vi "Replase ALR_ON_OFF.vi"(6 "Message":string, 8 "error in":errorcluster, 9 "Action":string, 10 "ALR_Names":string[](array[string]), 11 "Alarms_in":T1) -> (0 "error out":errorcluster, 3 "ALR_ON_OFF out":T1)   [LabVIEW 2019, in "Alarms.lvlib"]
uses:
  Alarms.lvlib
  Ctl/Alarms.ctl
  Ctl/ALR_defs.ctl
  Ctl/ALRs_State.ctl
  Ctl/ALR_ON_OFF.ctl
  Ctl/ALR_Parameters.ctl
  Ctl/ALR code.ctl
  Ctl/ALR type.ctl
  <vilib>/JDP Science/JSONtext/Find Multiple Items.vi
  <vilib>/JDP Science/JSONtext/String Subset.vi
  <vilib>/JDP Science/JSONtext/support/Strip Quotes and Unescape.vi
  <vilib>/JDP Science/JSONtext/Parsing/Parse Full Path or Item Name.vi
  <vilib>/JDP Science/JSONtext/Offset/Find Item Locations by Path.vi
  <vilib>/JDP Science/JSONtext/support/Unescape JSON string.vi
  <vilib>/JDP Science/JSONtext/Get Array Elements.vi
  Userlib.lvlib
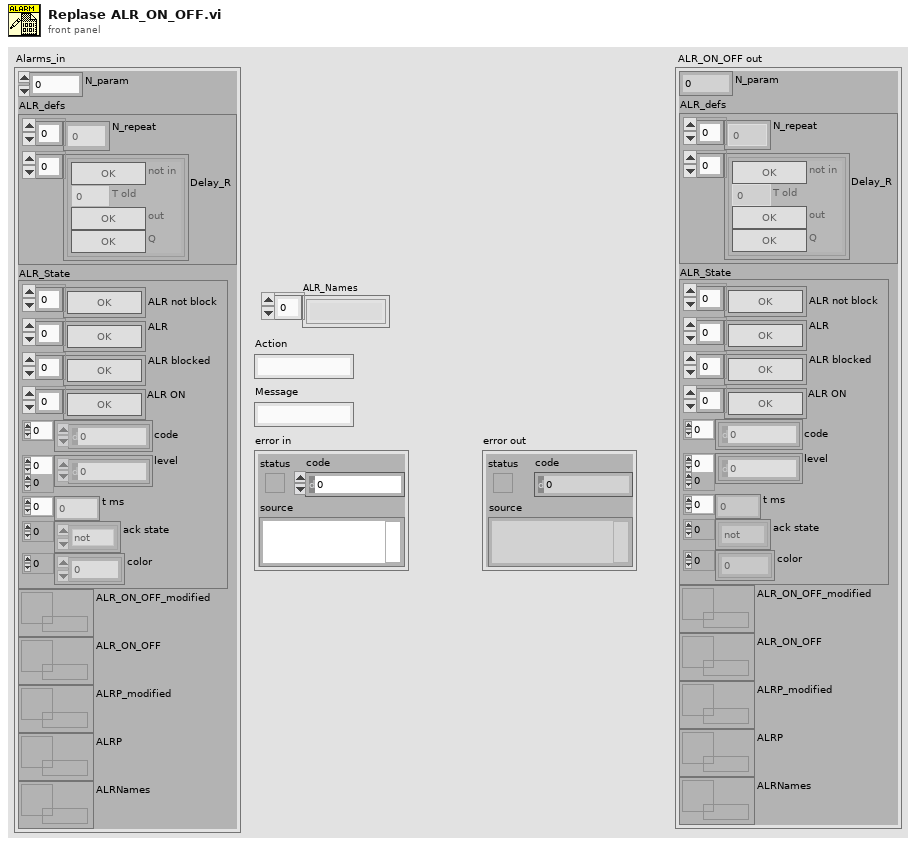
[diagram p1: front panel]
types:
  T1 = typedef "Alarms.lvlib/Alarms.ctl" = cluster{"N_param":i32, "ALR_defs":T2, "ALR_State":T3, "ALR_ON_OFF_modified":refnum<data-value>, "ALR_ON_OFF":refnum<data-value>, "ALRP_modified":refnum<data-value>, "ALRP":refnum<data-value>, "ALRNames":refnum<data-value>}
  T2 = typedef "Alarms.lvlib/ALR_defs.ctl" = cluster{"N_repeat":u32[], "Delay_R":cluster{"not in":bool, "T old":u32, "out":bool, "Q":bool}[]}
  T3 = typedef "Alarms.lvlib/ALRs_State.ctl" = cluster{"ALR not block":bool[], "ALR":bool[], "ALR blocked":bool[], "ALR ON":bool[], "code":i32[], "level":i32[][], "t ms":u32[], "ack state":enum32{"not", "tripped", "reset", "ack"}[], "color":u32[]}
  T4 = typedef "Alarms.lvlib/ALR_ON_OFF.ctl" = cluster{"ALR_ON":bool[], "ALR_OFF":bool[], "ALR_reset":bool[], "ALR_check":bool[], "ALR_block":bool[], "ALR_Ack":bool[]}
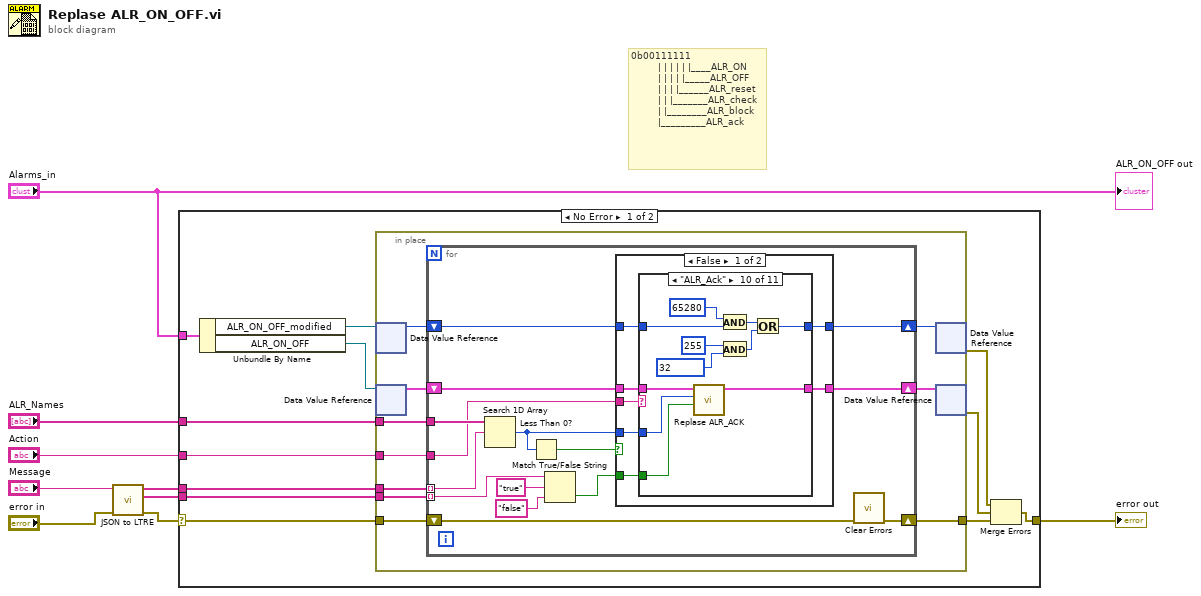
[diagram p0: block diagram]
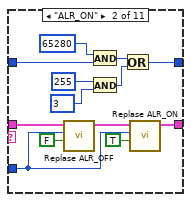
[diagram p3: hidden frame]
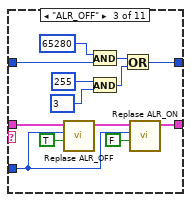
[diagram p4: hidden frame]
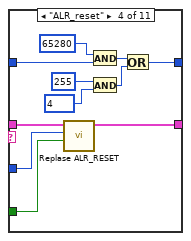
[diagram p5: hidden frame]
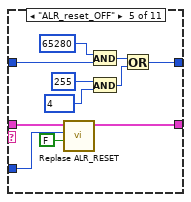
[diagram p6: hidden frame]
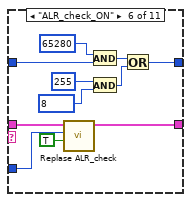
[diagram p7: hidden frame]
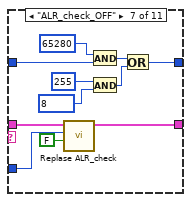
[diagram p8: hidden frame]
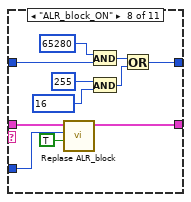
[diagram p9: hidden frame]
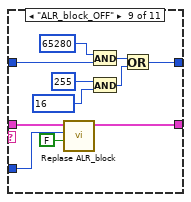
[diagram p10: hidden frame]
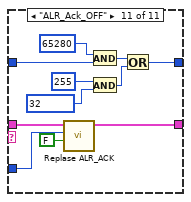
[diagram p11: hidden frame]
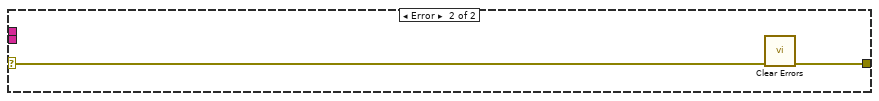
[diagram p13: hidden frame]
diagram:
  # "0b00111111\n         | | | | | |____ALR_ON\n         | | | | |_____ALR_OFF\n         | | | |______ALR_reset\n         | | |_______ALR_check\n         | |________ALR_block\n         |_________ALR_ack"
  n1 = call "JSON to LTRE.vi"("error in (no error)"="error in", "JSON Data In"="Message") -> ("error out"=w5:errorcluster, "values"=w4:string[], "names"=w3:string[])  [unwired: 7 in]
  n2 = case shown="No Error" w5 {
    selector: w5 -> [w21 w173]
    tunnel: w4 -> [w16 _]
    tunnel: [w18 w172] -> w9
    tunnel: w3 -> [w17 _]
    tunnel: "Action" -> [w15 _]
    tunnel: "Alarms_in" -> [w14 _]
    tunnel: "ALR_Names" -> [w11 _]
    frame No Error {
      n3 = Unbundle By Name(w14) -> ("ALR_ON_OFF_modified"=w13:refnum<data-value>, "ALR_ON_OFF"=w12:refnum<data-value>)
      n4 = in-place {
        in-place-border: w21 -> [w29]
        in-place-border: [w28] -> w19
        in-place-border: w17 -> [w27]
        in-place-border: w16 -> [w26]
        in-place-border: w15 -> [w25]
        in-place-border: w11 -> [w22]
        n5 = in-place-dvr #1(w13) -> (w24:u16)  [unwired: 1 out]
        n6 = in-place-dvr #2(w12) -> (w31:T4)  [unwired: 1 out]
        n7 = for {
          shift-right: [w45] -> w30
          shift-left: w31 -> [w46]
          tunnel: w27 -> [w44] mode=indexing
          tunnel: w22 -> [w43]
          tunnel: w26 -> [w34] mode=indexing
          shift-right: [w41] -> w28
          shift-left: w29 -> [w33]
          tunnel: w25 -> [w40]
          shift-right: [w38] -> w23
          shift-left: w24 -> [w39]
          n8 = Search 1D Array(1D array=w43, element=w44) -> (index of element=w42:i32)  [unwired: 1 in]
          n9 = Less Than 0?(x=w42) -> (x < 0?=w32:bool)
          n10 = Match True/False String(2:"false" ("false string"), 3:"true" ("true string"), 4:w34) -> (0:w35:bool)  [unwired: 1 out]
          n11 = case shown="False" w32 {
            tunnel: w46 -> [w53 w171]
            tunnel: [w52 w171] -> w45
            tunnel: w42 -> [w51 _]
            tunnel: w35 -> [w49 _]
            tunnel: w40 -> [w50 _]
            tunnel: w39 -> [w48 w170]
            tunnel: [w47 w170] -> w38
            frame False {
              n12 = case shown="\"ALR_Ack\"" w50 {
                tunnel: w53 -> [w55 w65 w79 w92 w103 w114 w125 w136 w147 w158 w169]
                tunnel: [w55 w68 w76 w91 w102 w113 w124 w135 w146 w157 w168] -> w52
                tunnel: w51 -> [_ w64 w78 w90 w100 w111 w122 w133 w144 w156 w166]
                tunnel: w49 -> [_ _ _ w89 _ _ _ _ _ w155 _]
                tunnel: w48 -> [w54 w56 w69 w83 w93 w104 w115 w126 w137 w149 w159]
                tunnel: [w54 w57 w70 w84 w94 w105 w116 w127 w138 w148 w160] -> w47
                frame "UNDEFINED", Default {
                }
                frame "ALR_ON" {
                  n13 = call "Replase ALR_OFF.vi"("ALR_OFF"=FALSE ("ALR_ON"), "N"=w64, "ALR_ON_OFF in"=w65) -> ("ALR_ON_OFF out"=w63:T4)  [unwired: 8 in]
                  n14 = And(x=u16 65280, y=w56) -> (x .and. y?=w62:u16)
                  n15 = And(x=u16 255, y=u16 3 ("modified (0)")) -> (x .and. y?=w61:u16)
                  n16 = Or(x=w62, y=w61) -> (x .or. y?=w57:u16)
                  n17 = call "Replase ALR_ON.vi"("ALR_ON"=TRUE, "N"=w64, "ALR_ON_OFF in"=w63) -> ("ALR_ON_OFF out"=w68:T4)  [unwired: 8 in]
                }
                frame "ALR_OFF" {
                  n18 = call "Replase ALR_OFF.vi"("ALR_OFF"=TRUE ("ALR_ON"), "N"=w78, "ALR_ON_OFF in"=w79) -> ("ALR_ON_OFF out"=w77:T4)  [unwired: 8 in]
                  n19 = And(x=u16 65280, y=w69) -> (x .and. y?=w75:u16)
                  n20 = And(x=u16 255, y=u16 3 ("modified (0)")) -> (x .and. y?=w74:u16)
                  n21 = Or(x=w75, y=w74) -> (x .or. y?=w70:u16)
                  n22 = call "Replase ALR_ON.vi"("ALR_ON"=FALSE, "N"=w78, "ALR_ON_OFF in"=w77) -> ("ALR_ON_OFF out"=w76:T4)  [unwired: 8 in]
                }
                frame "ALR_reset" {
                  n23 = call "Replase ALR_RESET.vi"("ALR_RST"=w89, "N"=w90, "ALR_ON_OFF in"=w92) -> ("ALR_ON_OFF out"=w91:T4)  [unwired: 8 in]
                  n24 = And(x=u16 65280, y=w83) -> (x .and. y?=w88:u16)
                  n25 = And(x=u16 255, y=u16 4 ("modified (0)")) -> (x .and. y?=w87:u16)
                  n26 = Or(x=w88, y=w87) -> (x .or. y?=w84:u16)
                }
                frame "ALR_reset_OFF" {
                  n27 = call "Replase ALR_RESET.vi"("ALR_RST"=FALSE, "N"=w100, "ALR_ON_OFF in"=w103) -> ("ALR_ON_OFF out"=w102:T4)  [unwired: 8 in]
                  n28 = And(x=u16 65280, y=w93) -> (x .and. y?=w99:u16)
                  n29 = And(x=u16 255, y=u16 4 ("modified (0)")) -> (x .and. y?=w98:u16)
                  n30 = Or(x=w99, y=w98) -> (x .or. y?=w94:u16)
                }
                frame "ALR_check_ON" {
                  n31 = call "Replase ALR_check.vi"("ALR_check"=TRUE, "N"=w111, "ALR_ON_OFF in"=w114) -> ("ALR_ON_OFF out"=w113:T4)  [unwired: 8 in]
                  n32 = And(x=u16 65280, y=w104) -> (x .and. y?=w110:u16)
                  n33 = And(x=u16 255, y=u16 8 ("modified (0)")) -> (x .and. y?=w109:u16)
                  n34 = Or(x=w110, y=w109) -> (x .or. y?=w105:u16)
                }
                frame "ALR_check_OFF" {
                  n35 = call "Replase ALR_check.vi"("ALR_check"=FALSE, "N"=w122, "ALR_ON_OFF in"=w125) -> ("ALR_ON_OFF out"=w124:T4)  [unwired: 8 in]
                  n36 = And(x=u16 65280, y=w115) -> (x .and. y?=w121:u16)
                  n37 = And(x=u16 255, y=u16 8 ("modified (0)")) -> (x .and. y?=w120:u16)
                  n38 = Or(x=w121, y=w120) -> (x .or. y?=w116:u16)
                }
                frame "ALR_block_ON" {
                  n39 = call "Replase ALR_block.vi"("ALR_block"=TRUE, "N"=w133, "ALR_ON_OFF in"=w136) -> ("ALR_ON_OFF out"=w135:T4)  [unwired: 8 in]
                  n40 = And(x=u16 65280, y=w126) -> (x .and. y?=w132:u16)
                  n41 = And(x=u16 255, y=u16 16 ("modified (0)")) -> (x .and. y?=w131:u16)
                  n42 = Or(x=w132, y=w131) -> (x .or. y?=w127:u16)
                }
                frame "ALR_block_OFF" {
                  n43 = call "Replase ALR_block.vi"("ALR_block"=FALSE ("ALR_check"), "N"=w144, "ALR_ON_OFF in"=w147) -> ("ALR_ON_OFF out"=w146:T4)  [unwired: 8 in]
                  n44 = And(x=u16 65280, y=w137) -> (x .and. y?=w143:u16)
                  n45 = And(x=u16 255, y=u16 16 ("modified (0)")) -> (x .and. y?=w142:u16)
                  n46 = Or(x=w143, y=w142) -> (x .or. y?=w138:u16)
                }
                frame "ALR_Ack" {
                  n47 = call "Replase ALR_ACK.vi"("ALR_ACK"=w155, "N"=w156, "ALR_ON_OFF in"=w158) -> ("ALR_ON_OFF out"=w157:T4)  [unwired: 8 in]
                  n48 = And(x=u16 65280, y=w149) -> (x .and. y?=w154:u16)
                  n49 = And(x=u16 255, y=u16 32 ("modified (0)")) -> (x .and. y?=w153:u16)
                  n50 = Or(x=w154, y=w153) -> (x .or. y?=w148:u16)
                }
                frame "ALR_Ack_OFF" {
                  n51 = call "Replase ALR_ACK.vi"("ALR_ACK"=FALSE, "N"=w166, "ALR_ON_OFF in"=w169) -> ("ALR_ON_OFF out"=w168:T4)  [unwired: 8 in]
                  n52 = And(x=u16 65280, y=w159) -> (x .and. y?=w165:u16)
                  n53 = And(x=u16 255, y=u16 32 ("modified (0)")) -> (x .and. y?=w164:u16)
                  n54 = Or(x=w165, y=w164) -> (x .or. y?=w160:u16)
                }
              }
            }
            frame True {
            }
          }
          n55 = call <vilib>:"Clear Errors.vi"("error in (no error)"=w33) -> ("error out"=w41:errorcluster)  [unwired: 5 in, 1 out]
        }
        n56 = in-place-dvr #1(w23) -> (w10:errorcluster)  [unwired: 1 out]
        n57 = in-place-dvr #2(w30) -> (w20:errorcluster)  [unwired: 1 out]
      }
      n58 = Merge Errors(w10, w20, w19) -> (w18:errorcluster)
    }
    frame Error {
      n59 = call <vilib>:"Clear Errors.vi"("error in (no error)"=w173) -> ("error out"=w172:errorcluster)  [unwired: 5 in, 1 out]
    }
  }
  "error out" <- w9
  "ALR_ON_OFF out" <- "Alarms_in"
